vi "Get Circus Logo.vi"() -> (0 "Circus Logo":picture)   [LabVIEW 2026, in "TALOS.lvlib"]
uses:
  TALOS.lvlib
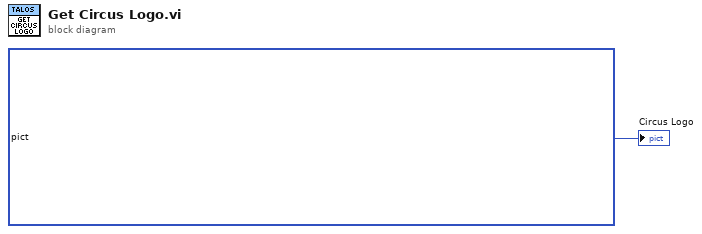
[diagram p0: block diagram]
diagram:
  "Circus Logo" <- picture bytes[327280] ("Circus Logo")
